vi "VI Server Control N2 Text In.vi"(1 "command text in":string[](array[string])) -> (0 "VI Server Control N2":T1={"VI name"="", "Control"=["1"], "Value"=[1.0], "Boolean?"=[1.0], "Wait Option"=enum."Wait Until", "wait (sec)"=5.0, "Control to End"="", "finish boolean?"=enum."not boolean", "Condition"=enum."within xxx% of target value", "Target Value"=20.0, "xxx%"=1.0, "update every (s)"=2.0, "Timeout (sec)"=3600.0} {"Boolean?" min=0.0 max=1.0 step=1.0 format="%#_1g"})   [LabVIEW 2024]
uses:
  VI Server Control N2.ctl
  condition.ctl
panel:
  # "Value of Control\n(if control is boolean type\n1 for \"ON\" and,0 for \"OFF\")"
  # "Is this control Boolean?\n(Yes: 1,  No: 0)"
  # "Name of  Control"
  # "0"
  # "1"
  # "2"
  # "3"
  # "4"
  # "5"
  # "6"
  # "7"
  # "8"
  # "9"
  # "1."
  # "Purely wait for"
  # "seconds"
  # "2."
  # "Control / Indicator Name"
  # "which is"
  # "Finish if"
  # "meets the following conditions"
  # "(check and update every"
  # "seconds)"
  # "3. Timeout"
  # "Wait until the following condition meets."
  # "Do not wait and move on to the next line in sequence."
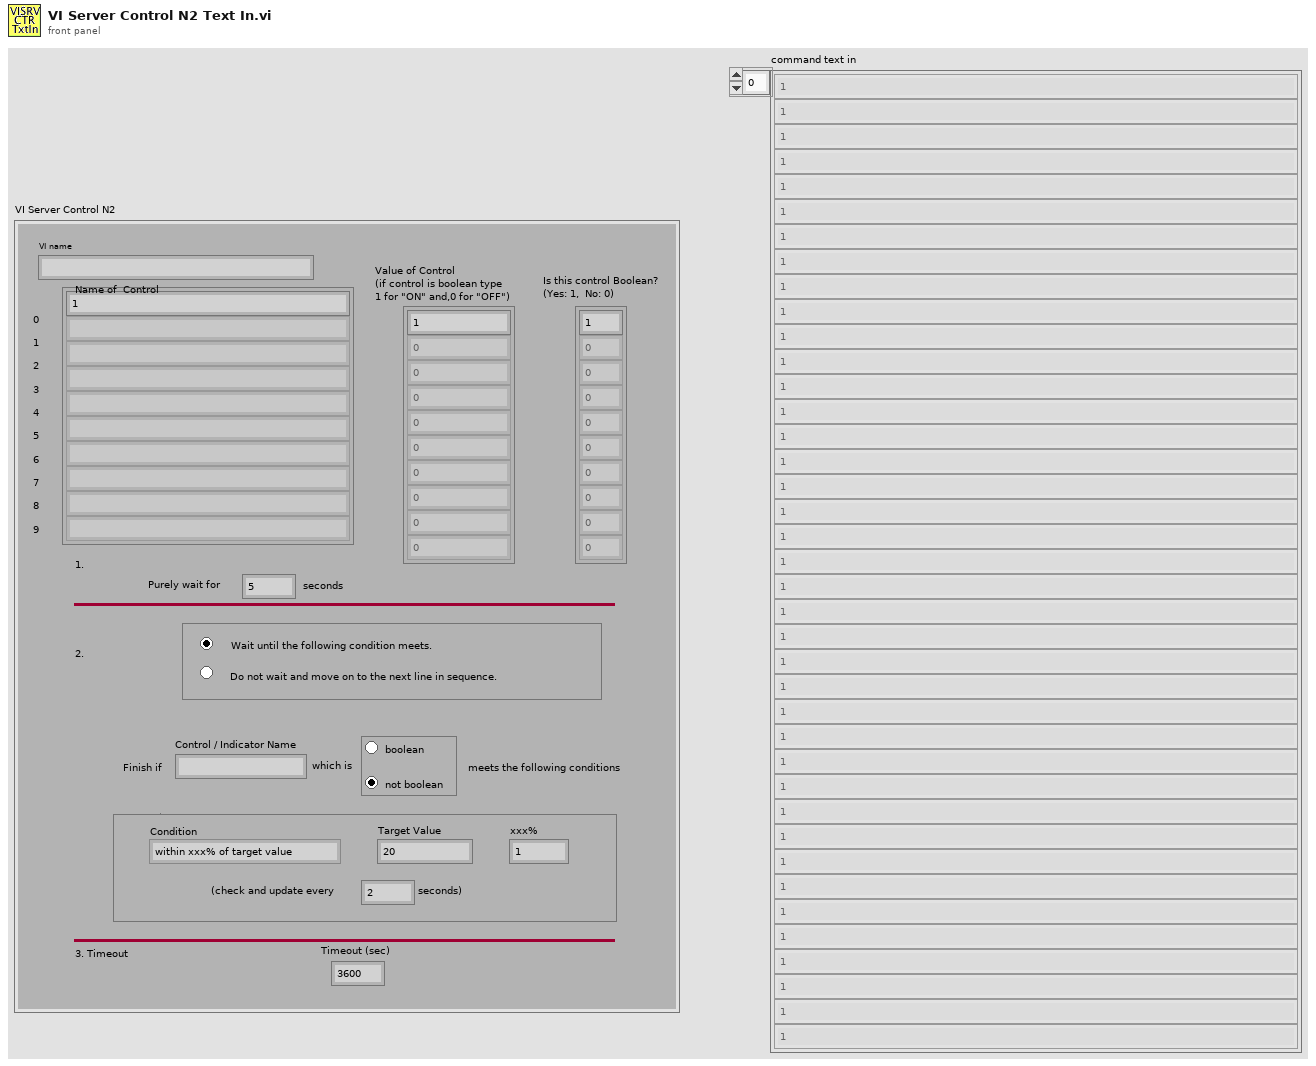
[diagram p1: front panel]
types:
  T1 = typedef "VI Server Control N2.ctl" = cluster{"VI name":string, "Control":string[], "Value":dbl[], "Boolean?":dbl[], "Wait Option":enum32{"Wait Until", "Do Not Wait"}, "wait (sec)":dbl, "Control to End":string, "finish boolean?":enum32{"boolean", "not boolean"}, "Condition":T2, "Target Value":dbl, "xxx%":dbl, "update every (s)":dbl, "Timeout (sec)":dbl}
  T2 = typedef "condition.ctl" = enum16{"within xxx% of target value", "<= target value", ">= target value", "= target value", "Boolean ON", "Boolean OFF"}
  T3 = cluster{"command text in[0]":string, "command text in[1]":string, "command text in[2]":string, "command text in[3]":string, "command text in[4]":string, "command text in[5]":string, "command text in[6]":string, "command text in[7]":string, "command text in[8]":string, "command text in[9]":string, "command text in[10]":string, "command text in[11]":string, "command text in[12]":string, "command text in[13]":string, "command text in[14]":string, "command text in[15]":string, "command text in[16]":string, "command text in[17]":string, "command text in[18]":string, "command text in[19]":string, "command text in[20]":string, "command text in[21]":string, "command text in[22]":string, "command text in[23]":string, "command text in[24]":string, "command text in[25]":string}
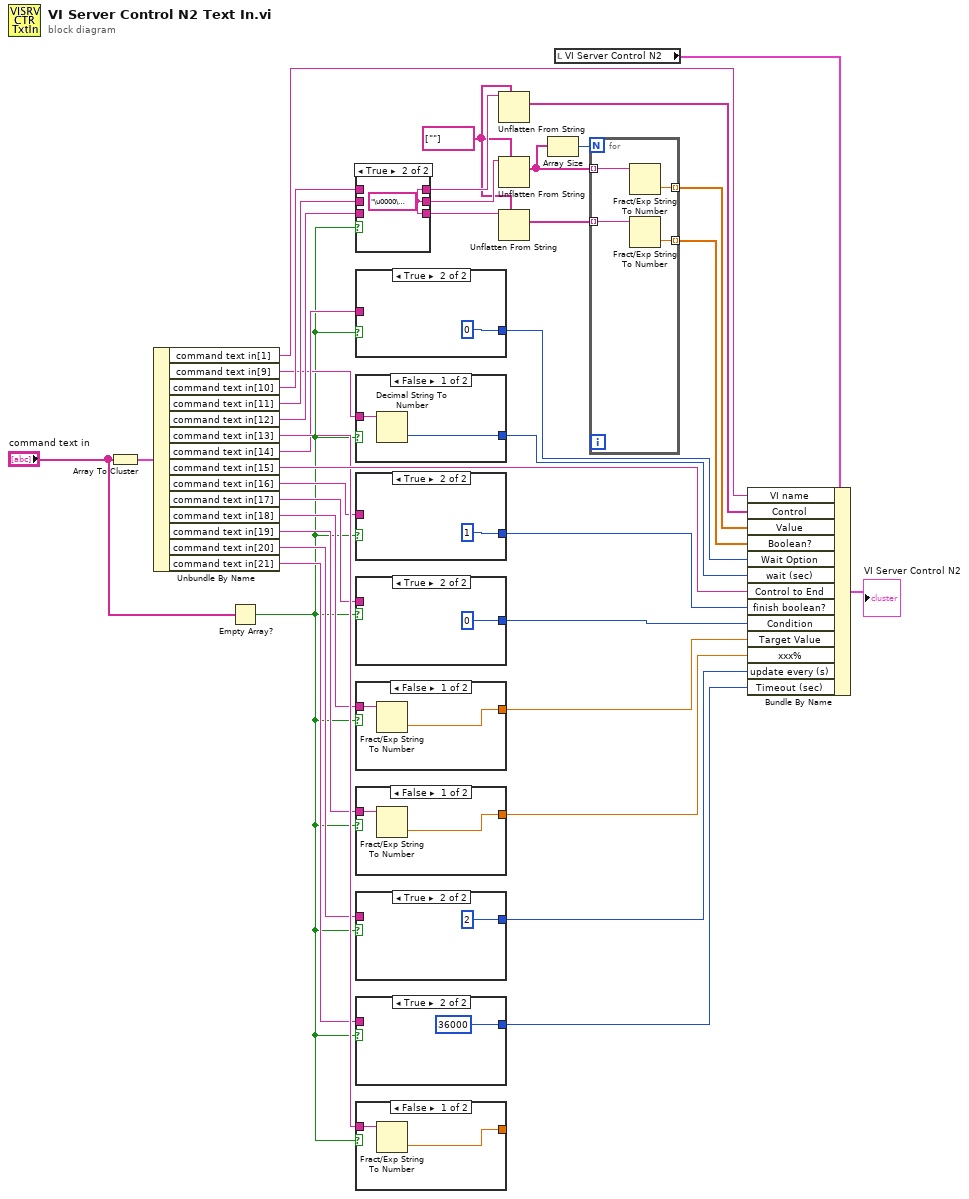
[diagram p0: block diagram]
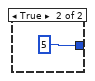
[diagram p2: hidden frame]
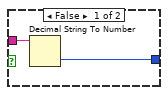
[diagram p3: hidden frame]
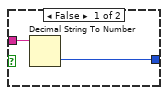
[diagram p4: hidden frame]
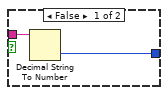
[diagram p5: hidden frame]
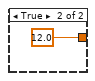
[diagram p6: hidden frame]
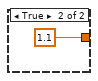
[diagram p7: hidden frame]
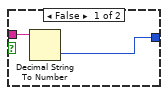
[diagram p8: hidden frame]
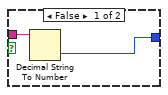
[diagram p9: hidden frame]
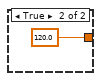
[diagram p10: hidden frame]
diagram:
  w20 = string[] [""] ("Control")
  n1 = Array To Cluster(array="command text in") -> (cluster=w35:T3)
  n2 = Unbundle By Name(w35) -> ("command text in[1]"=w34:string, "command text in[9]"=w2:string, "command text in[10]"=w29:string, "command text in[11]"=w28:string, "command text in[12]"=w27:string, "command text in[13]"=w18:string, "command text in[14]"=w5:string, "command text in[15]"=w33:string, "command text in[16]"=w6:string, "command text in[17]"=w8:string, "command text in[18]"=w11:string, "command text in[19]"=w13:string, "command text in[20]"=w15:string, "command text in[21]"=w16:string)
  n3 = Empty Array?(array="command text in") -> (empty?=w1:bool)
  n4 = case shown="True" w1 {
    tunnel: [w40 w41] -> w21
    tunnel: [w39 w41] -> w31
    tunnel: [w38 w41] -> w30
    tunnel: w29 -> [w40 _]
    tunnel: w28 -> [w39 _]
    tunnel: w27 -> [w38 _]
    frame False {
    }
    frame True {
      w41 = "\u0000\u0000\u0000\u0001\u0000\u0000\u0000\u00011" ("binary string")
    }
  }
  n5 = case shown="True" w1 {
    tunnel: w5 -> [w43 _]
    tunnel: [w42 0] -> w4
    frame False {
      n6 = Decimal String To Number(string=w43) -> (number=w42:i32)  [unwired: 2 in, 1 out]
    }
    frame True {
    }
  }
  n7 = case shown="False" w1 {
    tunnel: [w46 5] -> w3
    tunnel: w2 -> [w45 _]
    frame False {
      n8 = Decimal String To Number(string=w45) -> (number=w46:i32)  [unwired: 2 in, 1 out]
    }
    frame True {
    }
  }
  n9 = case shown="True" w1 {
    tunnel: w6 -> [w49 _]
    tunnel: [w48 1] -> w7
    frame False {
      n10 = Decimal String To Number(string=w49) -> (number=w48:i32)  [unwired: 2 in, 1 out]
    }
    frame True {
    }
  }
  n11 = case shown="True" w1 {
    tunnel: w8 -> [w52 _]
    tunnel: [w51 0] -> w9
    frame False {
      n12 = Decimal String To Number(string=w52) -> (number=w51:i32)  [unwired: 2 in, 1 out]
    }
    frame True {
    }
  }
  n13 = case shown="False" w1 {
    tunnel: w11 -> [w55 _]
    tunnel: [w54 12.0] -> w10
    frame False {
      n14 = Fract/Exp String To Number(string=w55) -> (number=w54:dbl)  [unwired: 3 in, 1 out]
    }
    frame True {
    }
  }
  n15 = case shown="False" w1 {
    tunnel: w13 -> [w58 _]
    tunnel: [w57 1.1] -> w12
    frame False {
      n16 = Fract/Exp String To Number(string=w58) -> (number=w57:dbl)  [unwired: 3 in, 1 out]
    }
    frame True {
    }
  }
  n17 = case shown="True" w1 {
    tunnel: w15 -> [w61 _]
    tunnel: [w60 2] -> w14
    frame False {
      n18 = Decimal String To Number(string=w61) -> (number=w60:i32)  [unwired: 2 in, 1 out]
    }
    frame True {
    }
  }
  n19 = case shown="True" w1 {
    tunnel: [w63 36000] -> w17
    tunnel: w16 -> [w64 _]
    frame False {
      n20 = Decimal String To Number(string=w64) -> (number=w63:i32)  [unwired: 2 in, 1 out]
    }
    frame True {
    }
  }
  n21 = case shown="False" w1 {
    tunnel: w18 -> [w67 _]
    tunnel: [w66 120.0] -> _
    frame False {
      n22 = Fract/Exp String To Number(string=w67) -> (number=w66:dbl)  [unwired: 3 in, 1 out]
    }
    frame True {
    }
  }
  n23 = Unflatten From String(type=w20, binary string=w21) -> (value=w19:string[])  [unwired: 3 in, 2 out]
  n24 = Unflatten From String(type=w20, binary string=w31) -> (value=w25:string[])  [unwired: 3 in, 2 out]
  n25 = Unflatten From String(type=w20, binary string=w30) -> (value=w23:string[])  [unwired: 3 in, 2 out]
  n26 = Array Size(array=w25) -> (size(s)=w26:i32)
  n27 = local read "VI Server Control N2"() -> (w36:T1)
  n28 = for {
    N: w26 -> [_]
    tunnel: w25 -> [w72] mode=indexing
    tunnel: [w71] -> w24 mode=indexing
    tunnel: w23 -> [w70] mode=indexing
    tunnel: [w69] -> w22 mode=indexing
    n29 = Fract/Exp String To Number(string=w72) -> (number=w71:dbl)  [unwired: 3 in, 1 out]
    n30 = Fract/Exp String To Number(string=w70) -> (number=w69:dbl)  [unwired: 3 in, 1 out]
  }
  n31 = Bundle By Name(cluster=w36, "VI name"=w34, "Control"=w19, "Value"=w24, "Boolean?"=w22, "Wait Option"=w4, "wait (sec)"=w3, "Control to End"=w33, "finish boolean?"=w7, "Condition"=w9, "Target Value"=w10, "xxx%"=w12, "update every (s)"=w14, "Timeout (sec)"=w17) -> (→"VI Server Control N2":T1)
